vi "close one relay channel.vi"(8 "error in (no error)":errorcluster caption="entrée d'erreur (pas d'erreur)", 10 "index":i32, 11 "hHandle":i32) -> (0 "error out":errorcluster caption="sortie d'erreur", 3 "function return":i32)   [LabVIEW 2020, in "usb_relay_device.lvlib"]
doc: "int EXPORT_API usb_relay_device_close_one_relay_channel(int hHandle, int index);"
uses:
  usb_relay_device.lvlib
  usb_relay_device.dll
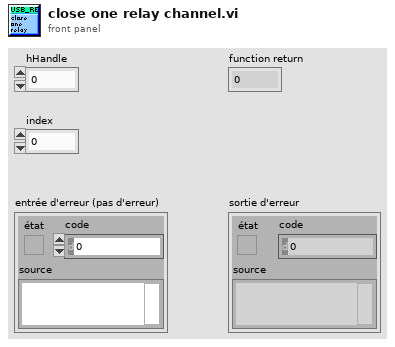
[diagram p1: front panel]
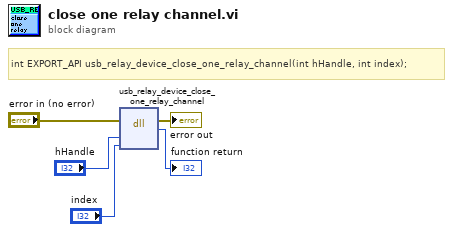
[diagram p0: block diagram]
diagram:
  # "int EXPORT_API usb_relay_device_close_one_relay_channel(int hHandle, int index);"
  n1 = dll-call lib="C:/Users/ngarcin/OneDrive - Altyor/Standard TB/Class/Relay_Board/Relay_Board usb_Relay_device/usb_relay_device/usb_relay_device.dll" fn="usb_relay_device_close_one_relay_channel"(error in="error in (no error)", "hHandle"="hHandle", "index"="index") -> (error out=→"error out":errorcluster, "type de retour"=→"function return":i32)  [unwired: 4 in, 1 out]
